vi "GetProperSampleRate.vi"(8 "error in (no error)":errorcluster, 10 "Sample Rate (0.00)":dbl format="%.2f", 11 "VISA Resource Name":refnum<visa-resource-name>) -> (0 "error out":errorcluster, 2 "New Sample Rate":dbl format="%.2f", 3 "VISA Resource Name Out":refnum<visa-resource-name>)   [LabVIEW 2010, in "Tektronix TDS 3000 Series.lvlib"]
doc: "Get's the proper value of the sample rate based on model."
uses:
  <instrlib>/Tektronix TDS 3000 Series/Tektronix TDS 3000 Series.lvlib
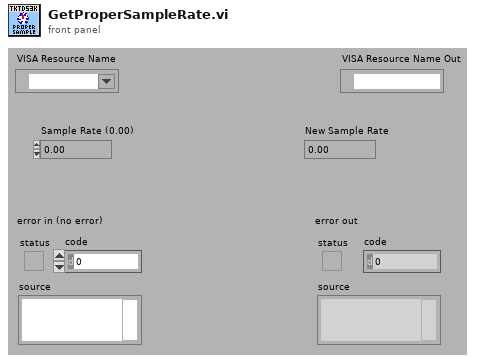
[diagram p1: front panel]
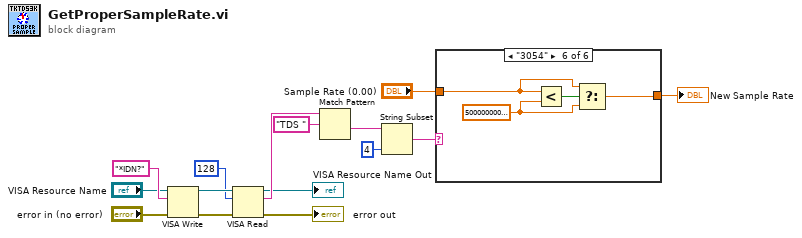
[diagram p0: block diagram]
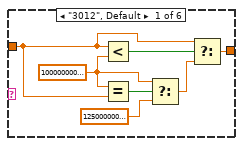
[diagram p2: hidden frame]
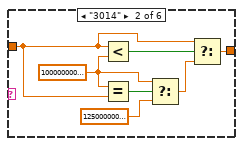
[diagram p3: hidden frame]
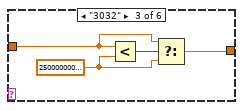
[diagram p4: hidden frame]
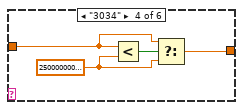
[diagram p5: hidden frame]
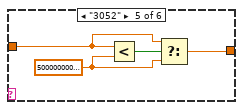
[diagram p6: hidden frame]
diagram:
  n1 = VISA Write(VISA resource name="VISA Resource Name", write buffer="*IDN?", error in (no error)="error in (no error)") -> (VISA resource name out=w15:refnum<visa-resource-name>, error out=w14:errorcluster)  [unwired: 1 out]
  n2 = VISA Read(VISA resource name=w15, byte count=u32 128, error in (no error)=w14) -> (VISA resource name out=→"VISA Resource Name Out":refnum<visa-resource-name>, read buffer=w11:string, error out=→"error out":errorcluster)  [unwired: 1 out]
  n3 = Match Pattern(string=w11, regular expression="TDS ") -> (after substring=w9:string)  [unwired: 1 in, 3 out]
  n4 = String Subset(string=w9, length (rest)=4 ("length (rest)")) -> (substring=w7:string)  [unwired: 1 in]
  n5 = case shown="\"3054\"" w7 {
    tunnel: "Sample Rate (0.00)" -> [w21 w28 w32 w36 w39 w43]
    tunnel: [w17 w24 w30 w34 w38 w42] -> w5
    frame "3012", Default {
      w16 = 1000000000.0 ("y")
      n6 = Less?(x=w21, y=w16) -> (x < y?=w22:bool)
      n7 = Equal?(x=w16, y=w21) -> (x = y?=w20:bool)
      n8 = Select(t=w16, s=w20, f=1250000000.0 ("y")) -> (s? t:f=w18:dbl)
      n9 = Select(t=w21, s=w22, f=w18) -> (s? t:f=w17:dbl)
    }
    frame "3014" {
      w23 = 1000000000.0 ("y")
      n10 = Less?(x=w28, y=w23) -> (x < y?=w29:bool)
      n11 = Equal?(x=w23, y=w28) -> (x = y?=w27:bool)
      n12 = Select(t=w23, s=w27, f=1250000000.0 ("y")) -> (s? t:f=w25:dbl)
      n13 = Select(t=w28, s=w29, f=w25) -> (s? t:f=w24:dbl)
    }
    frame "3032" {
      w31 = 2500000000.0 ("y")
      n14 = Less?(x=w32, y=w31) -> (x < y?=w33:bool)
      n15 = Select(t=w32, s=w33, f=w31) -> (s? t:f=w30:dbl)
    }
    frame "3034" {
      w35 = 2500000000.0 ("y")
      n16 = Less?(x=w36, y=w35) -> (x < y?=w37:bool)
      n17 = Select(t=w36, s=w37, f=w35) -> (s? t:f=w34:dbl)
    }
    frame "3052" {
      w40 = 5000000000.0 ("y")
      n18 = Less?(x=w39, y=w40) -> (x < y?=w41:bool)
      n19 = Select(t=w39, s=w41, f=w40) -> (s? t:f=w38:dbl)
    }
    frame "3054" {
      w44 = 5000000000.0 ("y")
      n20 = Less?(x=w43, y=w44) -> (x < y?=w45:bool)
      n21 = Select(t=w43, s=w45, f=w44) -> (s? t:f=w42:dbl)
    }
  }
  "New Sample Rate" <- w5
